vi "niFPGA I32xI32 Dot Product - 2 elements I64.vi"(0 "A[I32]":i32[](array[numeric])=[0, 0], 5 "B[I32]":i32[](array[numeric])=[0, 0]) -> (7 "A.B [I64]":i64=2838)   [LabVIEW 2017]
uses:
  <vilib>/Platform/TimedLoop/XDataNode/timing_clust.ctl
  <vilib>/Platform/TimedLoop/XDataNode/nitl_modes.ctl
  <vilib>/Platform/TimedLoop/XDataNode/wakeup.ctl
  <vilib>/Platform/TimedLoop/XDataNode/XDataNode.xnode
  <vilib>/Platform/TimedLoop/XDataNode/XDNodeRunTimeDep.lvlib
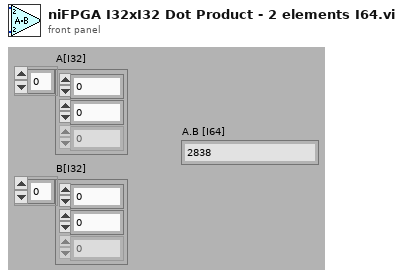
[diagram p1: front panel]
types:
  T1 = typedef "XDNodeRunTimeDep.lvlib/timing_clust.ctl" = cluster{"Expected End [f-1]":u64, "Actual End [f-1]":u64, "Finished Late? [f-1]":bool, "Expected End [i-1]":u64, "Actual End [i-1]":u64, "Finished Late? [i-1]":bool, "Expected Start [i]":u64, "Actual Start [i]":u64, "Expected Start [f]":u64, "Actual Start [f]":u64, "Source Name":string, "Structure Name":string, "Period":i64, "Deadline":i64, "Offset":i64, "Start":i64, "Priority":i32, "Timeout":i32, "Mode":T2, "Wakeup Reason":T3, "Error":errorcluster, "Source Type":string, "Secondary Source Type":string, "Global End Time":u64, "Global Start Time":u64, "Frame Duration":u64, "Iteration Duration":u64, "Assigned CPU":i32, "I/O Scan Engine Mode":u32}
  T2 = typedef "XDNodeRunTimeDep.lvlib/nitl_modes.ctl" = enum32{"No Change", "Process missed periods, maintain original phase", "Discard missed periods, maintain original phase", "Process missed periods, ignore original phase", "Discard missed periods, ignore original phase"}
  T3 = typedef "XDNodeRunTimeDep.lvlib/wakeup.ctl" = enum32{"Normal", "Aborted", "Asynchronous wakeup", "Timing source error", "Timed loop error", "Timeout"}
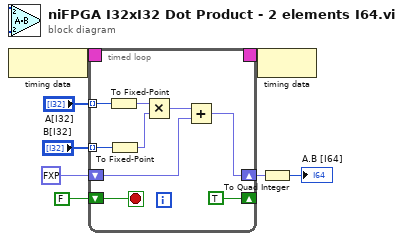
[diagram p0: block diagram]
diagram:
  n1 = node-c288() -> (w6:T1)
  n2 = timed-loop {
    shift-left: FALSE -> [w15]
    shift-right: [TRUE] -> _
    shift-left: fxp<+/-,64,64> 0.0 -> [w11]
    shift-right: [w17] -> w2
    tunnel: "A[I32]" -> [w14] mode=indexing
    tunnel: "B[I32]" -> [w13] mode=indexing
    timing: w6 -> [_]
    timing-out: [_] -> w5
    stop <- w15 stop-if-true
    n3 = To Fixed-Point(number=w14) -> (fixed-point=w10:fxp<+/-,32,32>)  [unwired: 1 out]
    n4 = To Fixed-Point(number=w13) -> (fixed-point=w9:fxp<+/-,32,32>)  [unwired: 1 out]
    n5 = Multiply(x=w10, y=w9) -> (x*y=w12:fxp<+/-,64,64>)
    n6 = Add(x=w12, y=w11) -> (x+y=w17:fxp<+/-,64,64>)
  }
  n7 = node-c288(w5) -> ()
  n8 = To Quad Integer(1:w2) -> (0:→"A.B [I64]":i64)
